vi "Read TX. Mode.vi"(8 "error in (no error)":errorcluster, 11 "Devices in":refnum<class "Devices.lvclass">) -> (0 "error out":errorcluster, 2 "TX. Mode":refnum<data-value>, 3 "Devices out":refnum<class "Devices.lvclass">)   [LabVIEW 2020, in "Devices.lvclass"]
uses:
  Devices.lvclass
  Transmission Mode/Parent/TX Speed.lvclass
  Devices.lvclass/Devices.ctl
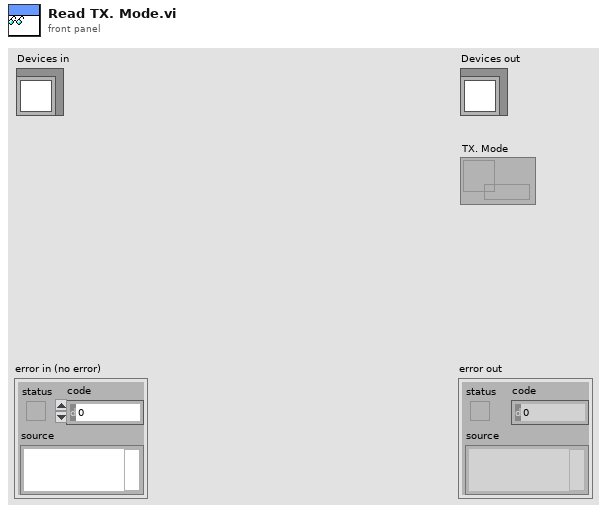
[diagram p1: front panel]
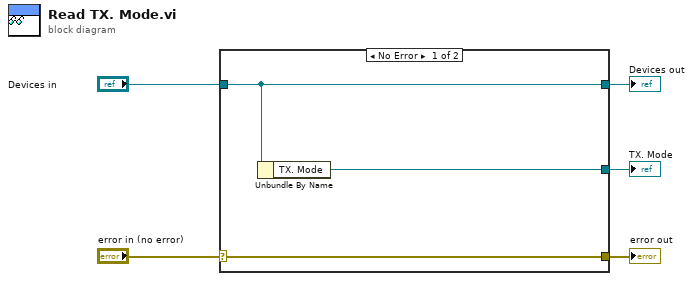
[diagram p0: block diagram]
diagram:
  n1 = case shown="No Error" "error in (no error)" {
    selector: "error in (no error)" -> [w8 w9]
    tunnel: [w8 w9] -> w4
    tunnel: [w7 w10] -> w2
    tunnel: "Devices in" -> [w7 w10]
    tunnel: [w6 _] -> w1
    frame No Error {
      n2 = Unbundle By Name(w7) -> ("TX. Mode"=w6:refnum<data-value>)
    }
    frame Error {
    }
  }
  "error out" <- w4
  "Devices out" <- w2
  "TX. Mode" <- w1
